vi "Simulate-Robot.vi"() -> ()   [LabVIEW 2023]
doc: "This VI implements the framework and scheduler for your robotics program. It should not be necessary to modify the framework. You are expected to add your code to the VIs called from Robot Main - the ones located in the Team Code folder within the project."
uses:
  <vilib>/Rock Robotics/WPI/DriverStation/WPI_DriverStationRobotMode2.ctl
  Climb/ClimbStates.ctl
  Intake/IntakeStates.ctl
  <vilib>/Rock Robotics/WPI/Camera/WPI_CameraImageSize.ctl
  <vilib>/Rock Robotics/WPI/ThirdParty/ADI/ADIS16470/Typedef/ADIS16470 Data.ctl
  <vilib>/Rock Robotics/WPI/ThirdParty/JAS_Junk/TrajLib/BatterySim_CalculateLoadedBatteryVoltage.vi
  Wrist/WristGlobal.vi
  Elevator/ElevatorGlobal.vi
  Robot Global Data.vi
  <vilib>/Rock Robotics/WPI/ThirdParty/JAS_Junk/TrajLib/Trajectory_Library.lvlib
panel:
  in  "Image Size":T1=enum."320x240"
  in  "Enable Vision":bool
  out "Voltage":dbl format="%13.1f"
  out "Motor Currents":dbl format="%13.1f"
  in  "Tab Control":T2(tab)
  out "Intake Chart":T3(graph)
  out "Intake Top Mot Dmd":dbl format="%9.2f"
  out "Intake Left Mot Dmd":dbl format="%9.1f"
  out "Intake Right Mot Dmd":dbl format="%9.1f"
  out "Intake State":T4
  out "Climb Chart":T3(graph)
  out "Climb Mot Dmd":dbl format="%9.2f"
  out "Climb Angle Deg":dbl format="%9.1f"
  out "Climb At Inner Limit":bool
  out "Climb At Outer Limit":bool
  out "ClimbStates":T5
  out "Wrist Chart":T3(graph)
  out "WristMotorDmd":dbl format="%9.2f"
  out "WristAngle Deg":dbl format="%9.1f"
  out "WristSP Deg":dbl format="%9.1f"
  out "Outer Elevator":T3(graph)
  out "Outer MotorOutDmd":dbl format="%9.2f"
  out "Outer HeightInch":dbl format="%9.1f"
  out "Outer Low Limit Switch":bool
  out "Outer HighLimitSwitch":bool
  out "Outer HeightSP_Inch":dbl format="%9.1f"
  out "Inner Elevator":T3(graph)
  out "Inner MotorOutDmd":dbl format="%9.2f"
  out "Inner HeightInch":dbl format="%9.1f"
  out "Inner Low Limit":bool
  out "Inner HighLimit":bool
  out "Inner HeightSP_Inch":dbl format="%9.1f"
  in  "Intake HaveAlgae":bool
  in  "Intake HaveCoral":bool
  out "Robot Mode":T6
  in  "Finish":bool
  # "Sensor Simulation"
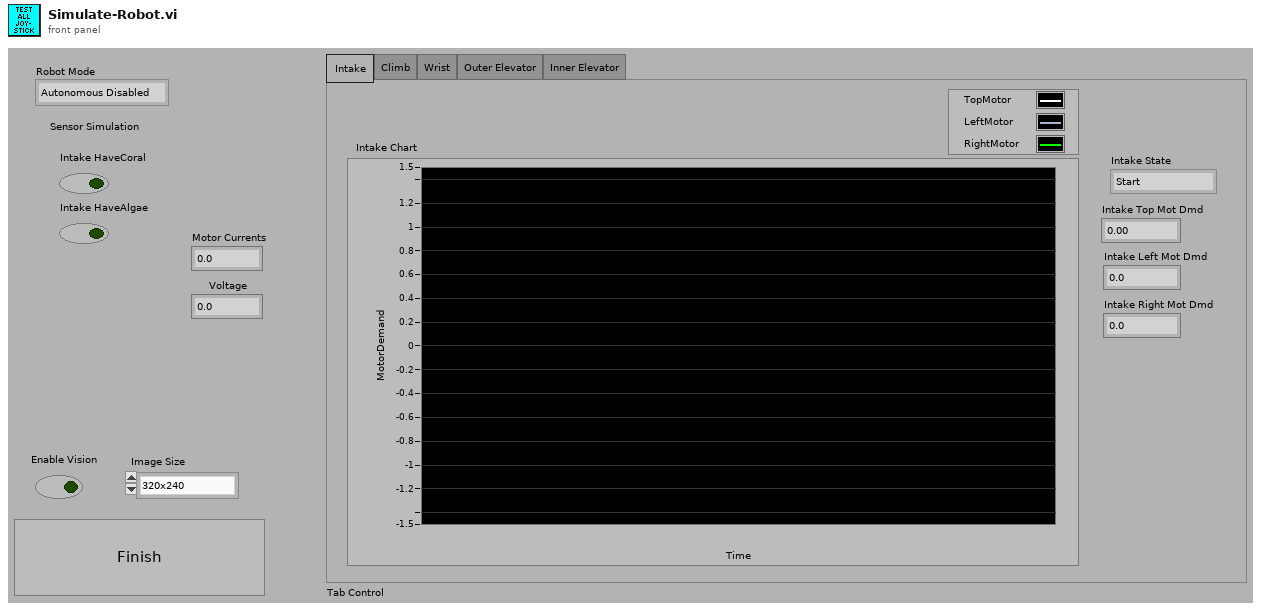
[diagram p1: front panel]
types:
  T1 = typedef "WPI_CameraImageSize.ctl" = enum16{"640x480", "320x240", "160x120", "Custom"}
  T2 = enum32{"Intake ", "Climb", "Wrist", "Outer Elevator", "Inner Elevator"}
  T3 = cluster{"ElevatorPosDemandHeight":dbl, "ElevHeightInch":dbl, "MotorDemand":dbl}
  T4 = typedef "IntakeStates.ctl" = enum16{"Start", "WaitForCommand", "IntakeCoral", "IntakeAlgae", "WaitForCoral", "WaitForAlgae", "DepositCoral", "DepositAlgae", "DepositCoralTimer", "DepositAlgaeTimer"}
  T5 = typedef "ClimbStates.ctl" = enum16{"Start", "WaitForCommands", "ClimbRest", "ClimbReach", "ClimbPull"}
  T6 = typedef "WPI_DriverStationRobotMode2.ctl" = enum16{"Autonomous Disabled", "Autonomous Enabled", "Teleop Disabled", "Teleop Enabled", "Disconnected", "Finish", "Test Disabled", "Test Enabled", "Emergency Stopped"}
  T7 = typedef "ADIS16470 Data.ctl" = cluster{"XAngle":dbl, "YAngle":dbl, "ZAngle":dbl}
  T8 = cluster{"MotorDemandTop":dbl, "MotorDemandLeft":dbl, "MotorDemandRight":dbl}
  T9 = typedef "Trajectory_Library.lvlib/SWERVE_DRIVE_MODULE_STATE.ctl" = cluster{"Speed":dbl, "Angle":T10}
  T10 = typedef "Trajectory_Library.lvlib/ROTATION2D.ctl" = cluster{"VALUE":dbl, "COS":dbl, "SIN":dbl}
  T11 = typedef "Trajectory_Library.lvlib/SWERVE_DRIVE_MODULE_POSITION.ctl" = cluster{"Distance":dbl, "Angle":T10, "P":bool}
  T12 = typedef "ADIS16470 Status.ctl" = cluster{"Calibrated?":bool, "IMU Detected?":bool}
  T13 = typedef "Trajectory_Library.lvlib/SWERVE_DRIVE_KINEMATICS.ctl" = cluster{"NumModules":i32, "InverseKinematics":T14, "ForwardKinematics":T14, "Modules":T15[], "PrevCoR":T15, "SavedModuleStates":T9[]}
  T14 = typedef "NI_Matrix.lvlib/RealMatrix.ctl" = dbl[][]
  T15 = typedef "Trajectory_Library.lvlib/TRANSLATION2D.ctl" = cluster{"X":dbl, "Y":dbl}
  T16 = cluster{"WristSP Deg 2":dbl, "ClimbPositionDegrees":dbl, "MotorDemand":dbl}
  T17 = cluster{"ElevatorStage3PosDemandHeight":dbl, "Inner  HeightInches":dbl, "Stage3MotorDemand":dbl}
  T18 = cluster{"ElevatorOuterPosDemandHeight":dbl, "Outer ElevHeightInch":dbl, "OuterMotorDemand":dbl}
  T19 = cluster{"CurrentWristSetpoint":dbl, "WritstPositionDegrees":dbl, "MotorDmd":dbl}
  T20 = typedef "WPI_DriverStationMatch Info.ctl" = cluster{"Autonomous Elapsed Seconds":dbl, "TeleOp Elapsed Seconds":dbl, "Disabled Elapsed Seconds":dbl, "Visited Autonomous":bool, "Visited TeleOp":bool, "Visited Disabled":bool, "Autonomous Settings":cluster{"Autonomous Style":enum16{"Iterative", "Independent"}, "VI Refnum":refnum<vi>}}
  T21 = typedef "WPI_DriverStationDerivedRobotMode.ctl" = enum16{"Init", "Execute", "Stop"}
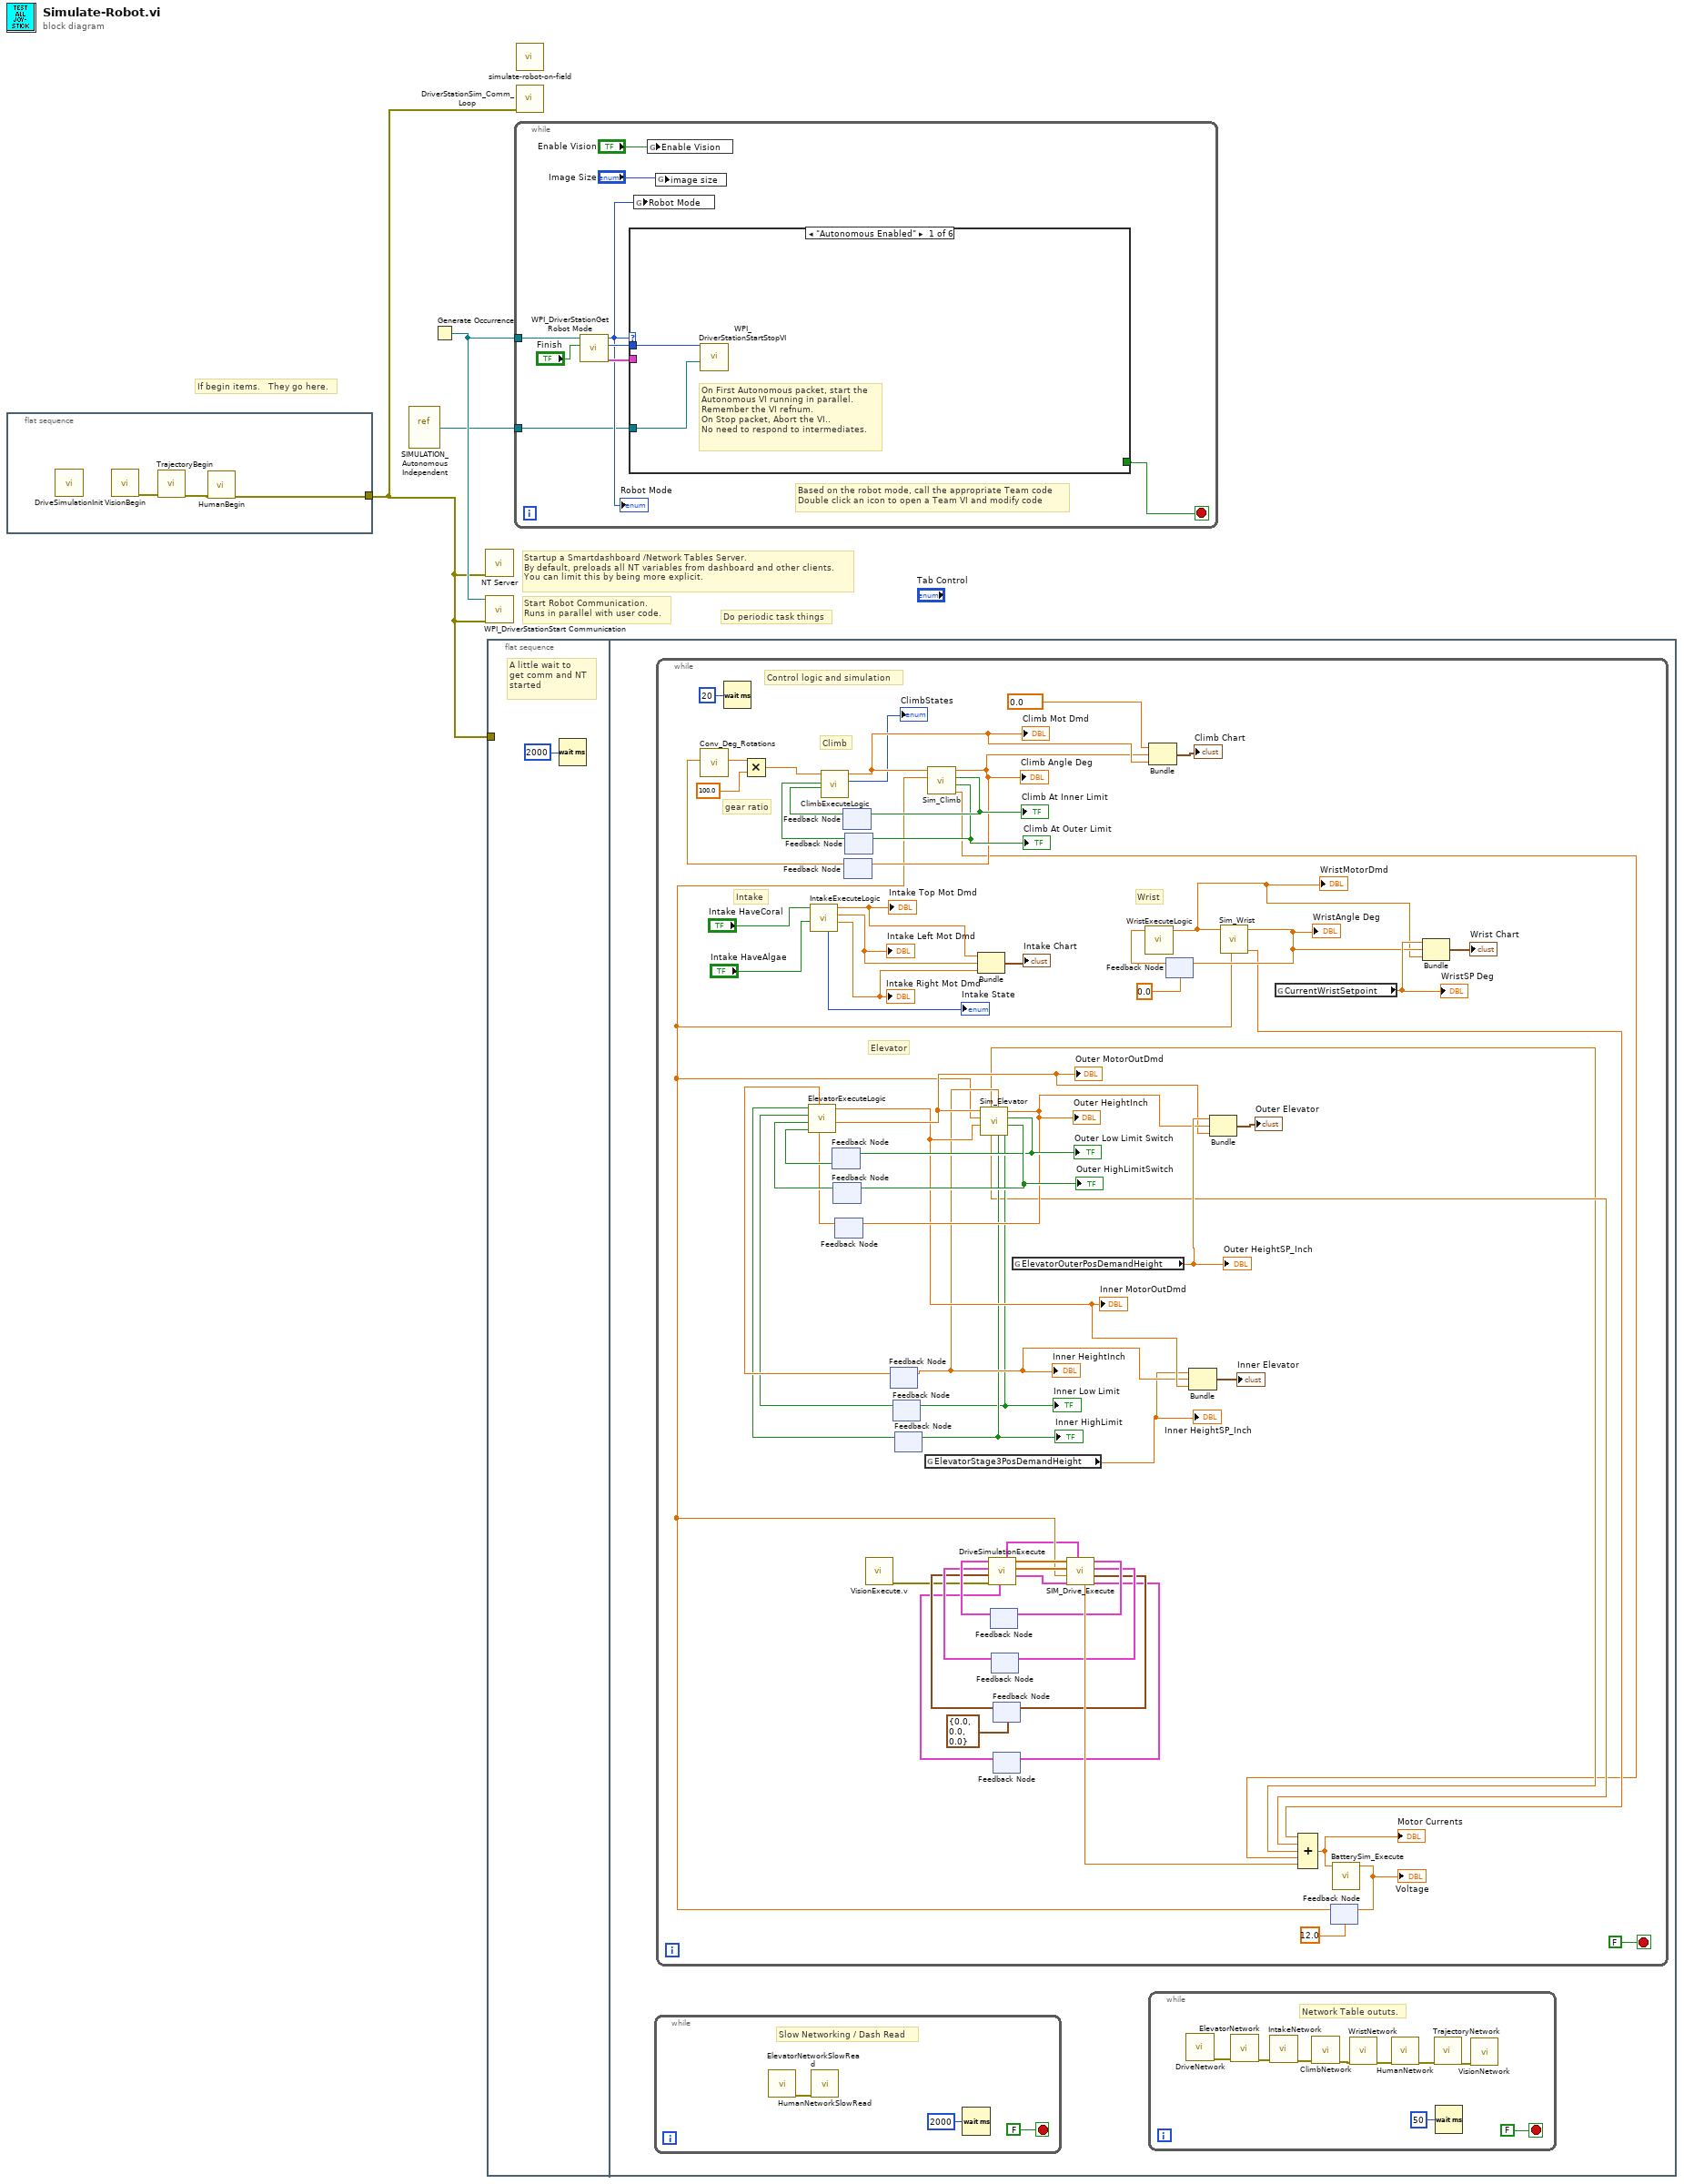
[diagram p0: block diagram]
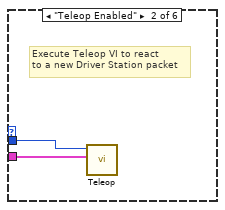
[diagram p2: hidden frame]
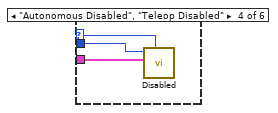
[diagram p4: hidden frame]
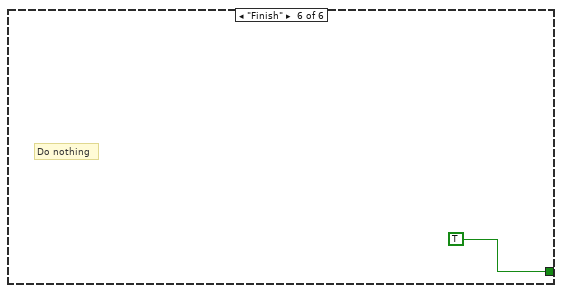
[diagram p6: hidden frame]
diagram:
  # "If begin items.   They go here."
  # "Do periodic task things"
  # "Startup a Smartdashboard /Network Tables Server.\nBy default, preloads all NT variables from dashboard and other clients.\nYou can limit this by being more explicit."
  # "Start Robot Communication.\nRuns in parallel with user code."
  n1 = flat-sequence {
    tunnel: [w6] -> w2
    frame #0 {
      n2 = call "DriveSimulationInit.vi"() -> ()  [unwired: 9 in, 3 out]
      n3 = call "VisionBegin.vi"() -> ("error out"=w4:errorcluster)  [unwired: 11 in]
      n4 = call "TrajectoryBegin.vi"("error in (no error)"=w4) -> ("error out"=w5:errorcluster)  [unwired: 10 in]
      n5 = call "HumanBegin.vi"("error in (no error)"=w5) -> ("error out"=w6:errorcluster)  [unwired: 10 in]
    }
  }
  n6 = vi-ref "SIMULATION_Autonomous Independent.vi"() -> (w1:refnum<vi>)
  n7 = Generate Occurrence() -> (w3:refnum<k4>)
  n8 = call <vilib>:"NT Server.vi"("error in (no error)"=w2) -> ()  [unwired: 10 in, 1 out]
  n9 = call <vilib>:"WPI_DriverStationStart Communication.vi"("error in (no error)"=w2, "occurrence"=w3) -> ()  [unwired: 1 in, 9 out]
  n10 = flat-sequence {
    tunnel: w2 -> [_]
    frame #0 {
      # "A little wait to\nget comm and NT\nstarted"
      n11 = Wait (ms)(milliseconds to wait=u32 2000) -> ()  [unwired: 1 out]
    }
    frame #1 {
      n12 = while {
        stop <- FALSE stop-if-true
        # "Slow Networking / Dash Read"
        n13 = call "ElevatorNetworkSlowRead.vi"() -> ("error out"=w8:errorcluster)  [unwired: 11 in]
        n14 = call "HumanNetworkSlowRead.vi"("error in (no error)"=w8) -> ()  [unwired: 10 in, 1 out]
        n15 = Wait (ms)(milliseconds to wait=u32 2000) -> ()  [unwired: 1 out]
      }
      n16 = while {
        stop <- FALSE stop-if-true
        # "Elevator"
        # "Wrist"
        # "Intake"
        # "gear ratio"
        # "Climb"
        # "Control logic and simulation"
        n17 = Wait (ms)(milliseconds to wait=u32 20) -> ()  [unwired: 1 out]
        n18 = call "IntakeExecuteLogic.vi"("HaveAlgaeSensor"="Intake HaveAlgae", "HaveCoralSensor"="Intake HaveCoral") -> ("MotorDemandRight"=w69:dbl, "MotorDemandLeft"=w70:dbl, "MotorDemandTop"=w71:dbl, "CurrentState"=→"Intake State":T4)  [unwired: 6 in]
        "Intake Top Mot Dmd" <- w71
        "Intake Left Mot Dmd" <- w70
        "Intake Right Mot Dmd" <- w69
        n19 = feedback #1() -> (w55:bool)  [unwired: 1 in]
        n20 = feedback #2() -> (w54:bool)  [unwired: 1 in]
        n21 = feedback #3() -> (w53:dbl)  [unwired: 1 in]
        n22 = feedback #4() -> (w77:bool)  [unwired: 1 in]
        n23 = feedback #5() -> (w78:dbl)  [unwired: 1 in]
        n24 = call <vilib>:"Conv_Deg_Rotations.vi"("Degrees"=w78) -> ("Rotations"=w81:dbl)  [unwired: 10 in]
        n25 = Multiply(x=w81, y=100.0) -> (x*y=w74:dbl)
        n26 = feedback #6() -> (w76:bool)  [unwired: 1 in]
        n27 = call "ClimbExecuteLogic.vi"("PullLS"=w77, "ReachLS"=w76, "SensorPosition"=w74) -> ("ClimbStates"=→"ClimbStates":T5, "MotorDemand"=w84:dbl)  [unwired: 6 in, 1 out]
        "Climb Mot Dmd" <- w84
        n28 = call "VisionExecute.v.vi"() -> ("error out"=w23:errorcluster)  [unwired: 11 in]
        n29 = feedback #7() -> (w51:dbl)  [unwired: 1 in]
        n30 = feedback #8() -> (w43:bool)  [unwired: 1 in]
        n31 = feedback #9() -> (w45:bool)  [unwired: 1 in]
        n32 = call "ElevatorExecuteLogic.vi"("OuterPositionHeight"=w53, "InnerPositionHeight"=w51, "OuterLowLimitSwitch"=w55, "OuterHighLimitSwitch"=w54, "Stage3LowLimitSwitch"=w43, "Stage3HighLimitSwitch"=w45) -> ("OuterMotorDemand"=w52:dbl, "Stage3MotorDemand"=w50:dbl)  [unwired: 4 in]
        "Outer MotorOutDmd" <- w52
        "Inner MotorOutDmd" <- w50
        n33 = global read "ElevatorGlobal.vi" "ElevatorStage3PosDemandHeight"() -> (w48:dbl)
        "Inner HeightSP_Inch" <- w48
        n34 = Bundle("MotorDemandTop"=w71, "MotorDemandLeft"=w70, "MotorDemandRight"=w69) -> (→"Intake Chart":T8)  [unwired: 1 in]
        n35 = feedback #10() -> (w30:T9[])  [unwired: 1 in]
        n36 = feedback #11() -> (w28:T11[])  [unwired: 1 in]
        n37 = feedback #12(T7 {"XAngle"=0.0, "YAngle"=0.0, "ZAngle"=0.0} ("GyroValuesDeg")) -> (w26:T7)
        n38 = feedback #13() -> (w24:T12)  [unwired: 1 in]
        n39 = call "DriveSimulationExecute.vi"("GyroStatus"=w24, "error in (no error)"=w23, "GyroValuesDeg"=w26, "ModulePositions"=w28, "ModuleStates"=w30) -> ("outModulePositions"=w21:T11[], "SpinMotorDmds"=w34:dbl[], "TravelMotorDmds"=w35:dbl[], "out SWERVE_DRIVE_KINEMATICS"=w22:T13)  [unwired: 2 in, 1 out]
        n40 = global read "ElevatorGlobal.vi" "ElevatorOuterPosDemandHeight"() -> (w58:dbl)
        "Outer HeightSP_Inch" <- w58
        n41 = feedback #14(0.0 ("WritstPositionDegrees")) -> (w65:dbl)
        n42 = call "WristExecuteLogic.vi"("EncoderPos (deg)"=w65) -> ("MotorDmd"=w61:dbl)  [unwired: 9 in, 1 out]
        "WristMotorDmd" <- w61
        n43 = global read "WristGlobal.vi" "CurrentWristSetpoint"() -> (w64:dbl)
        "WristSP Deg" <- w64
        n44 = feedback #15(12.0 ("Voltage")) -> (w33:dbl)
        n45 = call "Sim_Climb.vi"("Battery Volts"=w33, "Motor1 Dmd"=w84) -> ("Motor Current"=w36:dbl, "At Outer Limit"=w82:bool, "At Climbed Limit"=w83:bool, "ClimbPositionDegrees"=w79:dbl)  [unwired: 6 in]
        "Climb Angle Deg" <- w79
        "Climb At Inner Limit" <- w83
        "Climb At Outer Limit" <- w82
        n46 = feedback-in #4(w83) -> ()
        n47 = feedback-in #5(w79) -> ()
        n48 = feedback-in #6(w82) -> ()
        n49 = call "Sim_Elevator.vi"("Inner Demand"=w50, "Battery Voltage"=w33, "Outer Dmd"=w52) -> ("Inner At Low Limit"=w44:bool, "OuterHighLimitSwitch"=w60:bool, "Outer Low Limit Switch"=w59:bool, "Outer ElevHeightInch"=w57:dbl, "Inner At High Limit"=w46:bool, "Inner  HeightInches"=w49:dbl, "Inner Current"=w38:dbl, "Outer Current"=w37:dbl)  [unwired: 1 in]
        "Outer HeightInch" <- w57
        "Outer Low Limit Switch" <- w59
        "Outer HighLimitSwitch" <- w60
        "Inner HeightInch" <- w49
        "Inner Low Limit" <- w44
        "Inner HighLimit" <- w46
        n50 = feedback-in #1(w59) -> ()
        n51 = feedback-in #2(w60) -> ()
        n52 = feedback-in #3(w57) -> ()
        n53 = feedback-in #7(w49) -> ()
        n54 = feedback-in #8(w44) -> ()
        n55 = feedback-in #9(w46) -> ()
        n56 = call "SIM_Drive_Execute.vi"("SwerveKinematics"=w22, "in Module Positions"=w21, "Battery Voltage"=w33, "SpinMotorDmds"=w34, "TravelMotorDmds"=w35) -> ("GyroStatus"=w25:T12, "GyroValuesDeg"=w27:T7, "out ModulePositions"=w29:T11[], "ModuleStates"=w31:T9[], "Motor Currents"=w32:dbl)  [unwired: 2 in]
        n57 = feedback-in #10(w31) -> ()
        n58 = feedback-in #11(w29) -> ()
        n59 = feedback-in #12(w27) -> ()
        n60 = feedback-in #13(w25) -> ()
        n61 = Bundle("WristSP Deg 2"=0.0, "ClimbPositionDegrees"=w79, "MotorDemand"=w84) -> (→"Climb Chart":T16)  [unwired: 1 in]
        n62 = Bundle("ElevatorStage3PosDemandHeight"=w48, "Inner  HeightInches"=w49, "Stage3MotorDemand"=w50) -> (→"Inner Elevator":T17)  [unwired: 1 in]
        n63 = Bundle("ElevatorOuterPosDemandHeight"=w58, "Outer ElevHeightInch"=w57, "OuterMotorDemand"=w52) -> (→"Outer Elevator":T18)  [unwired: 1 in]
        n64 = call "Sim_Wrist.vi"("Battery Voltage"=w33, "Motor1 Dmd"=w61) -> ("Motor Current"=w39:dbl, "WritstPositionDegrees"=w63:dbl)  [unwired: 6 in, 2 out]
        "WristAngle Deg" <- w63
        n65 = feedback-in #14(w63) -> ()
        n66 = Compound Arithmetic op=ADD(w39, w38, w37, w36, w32) -> (w40:dbl)
        "Motor Currents" <- w40
        n67 = call <vilib>:"BatterySim_Execute.vi"("Current"=w40) -> ("Voltage"=w42:dbl)  [unwired: 10 in]
        "Voltage" <- w42
        n68 = feedback-in #15(w42) -> ()
        n69 = Bundle("CurrentWristSetpoint"=w64, "WritstPositionDegrees"=w63, "MotorDmd"=w61) -> (→"Wrist Chart":T19)  [unwired: 1 in]
      }
      n70 = while {
        stop <- FALSE stop-if-true
        # "Network Table oututs."
        n71 = call "DriveNetwork.vi"() -> ("error out"=w13:errorcluster)  [unwired: 11 in]
        n72 = call "ElevatorNetwork.vi"("error in (no error)"=w13) -> ("error out"=w17:errorcluster)  [unwired: 10 in]
        n73 = call "IntakeNetwork.vi"("error in (no error)"=w17) -> ("error out"=w16:errorcluster)  [unwired: 10 in]
        n74 = call "ClimbNetwork.vi"("error in (no error)"=w16) -> ("error out"=w15:errorcluster)  [unwired: 10 in]
        n75 = call "WristNetwork.vi"("error in (no error)"=w15) -> ("error out"=w14:errorcluster)  [unwired: 10 in]
        n76 = call "HumanNetwork.vi"("error in (no error)"=w14) -> ("error out"=w11:errorcluster)  [unwired: 10 in]
        n77 = call "TrajectoryNetwork.vi"("error in (no error)"=w11) -> ("error out"=w12:errorcluster)  [unwired: 10 in]
        n78 = Wait (ms)(milliseconds to wait=u32 50) -> ()  [unwired: 1 out]
        n79 = call "VisionNetwork.vi"("error in (no error)"=w12) -> ()  [unwired: 10 in, 1 out]
      }
    }
  }
  n80 = while {
    tunnel: w3 -> [w97]
    tunnel: w1 -> [w89]
    stop <- w92 stop-if-true
    # "Based on the robot mode, call the appropriate Team code\nDouble click an icon to open a Team VI and modify code"
    n81 = call <vilib>:"WPI_DriverStationGet Robot Mode.vi"("Finish"="Finish", "DS Occurrence"=w97) -> ("Match Info out"=w94:T20, "Call Context"=w96:T21, "Robot Mode"=w93:T6)  [unwired: 7 out]
    "Robot Mode" <- w93
    n82 = case shown="\"Autonomous Enabled\"" w93 {
      selector: w93 -> [_ _ _ w104 _ _]
      tunnel: w96 -> [w99 w101 _ w103 _ _]
      tunnel: w94 -> [_ w100 _ w102 _ _]
      tunnel: [_ _ _ _ _ TRUE] -> w92
      tunnel: w89 -> [w98 _ _ _ _ _]
      frame "Autonomous Enabled" {
        # "On First Autonomous packet, start the\nAutonomous VI running in parallel.\nRemember the VI refnum.\nOn Stop packet, Abort the VI..\nNo need to respond to intermediates."
        n83 = call <vilib>:"WPI_DriverStationStartStopVI.vi"("VI in"=w98, "Call Context"=w99) -> ()  [unwired: 10 in]
      }
      frame "Teleop Enabled" {
        # "Execute Teleop VI to react\nto a new Driver Station packet"
        n84 = call "Teleop.vi"("Match Info"=w100, "Call Context"=w101) -> ()  [unwired: 1 in, 9 out]
      }
      frame "Test Disabled", "Test Enabled" {
        # "#NOTE FOR NOW TEST IS NOT SUPPORTED IN SIMULATION"
      }
      frame "Autonomous Disabled", "Teleop Disabled" {
        n85 = call "Disabled.vi"("Robot Mode"=w104, "Match Info"=w102, "Call Context"=w103) -> ()  [unwired: 1 in, 8 out]
      }
      frame "Disconnected", Default {
        # "Driver Station packet didn't arrive.\nPossibly useful for diagnostics"
      }
      frame "Finish" {
        # "Do nothing"
      }
    }
    n86 = global write "Robot Global Data.vi" "Robot Mode"(w93) -> ()
    n87 = global write "Robot Global Data.vi" "Enable Vision"("Enable Vision") -> ()
    n88 = global write "Robot Global Data.vi" "image size"("Image Size") -> ()
  }
  n89 = call "simulate-robot-on-field.vi"() -> ()  [unwired: 12 in]
  n90 = call <vilib>:"DriverStationSim_Comm_Loop.vi"("error in (no error)"=w2) -> ()  [unwired: 11 in]
